vi "Teleop.vi"(10 "Match Info":T1={"Autonomous Elapsed Seconds"=0.0, "TeleOp Elapsed Seconds"=0.0, "Disabled Elapsed Seconds"=0.0, "Visited Autonomous"=FALSE, "Visited TeleOp"=FALSE, "Visited Disabled"=FALSE, "Autonomous Settings"={"Autonomous Style"=enum."Independent", "VI Refnum"=refnum}}, 11 "Call Context":T2) -> ()   [LabVIEW 2011]
doc: "This VI is called for each TeleOp packet received from the DS where the robot is not disabled. It is often used to read from the joysticks and update I/O or to update setpoints for timed control loops. It should complete and return within 20 milliseconds or it may miss DS packets."
uses:
  <vilib>/Rock Robotics/WPI/DriverStation/WPI_DriverStationDerivedRobotMode.ctl
  <vilib>/Rock Robotics/WPI/DriverStation/WPI_DriverStationMatch Info.ctl
  Robot Global Data.vi
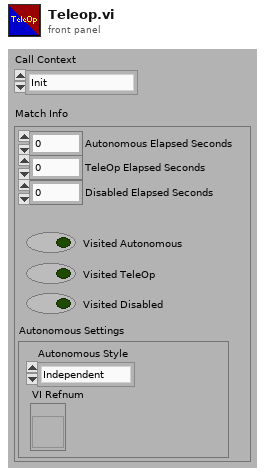
[diagram p1: front panel]
types:
  T1 = typedef "WPI_DriverStationMatch Info.ctl" = cluster{"Autonomous Elapsed Seconds":dbl, "TeleOp Elapsed Seconds":dbl, "Disabled Elapsed Seconds":dbl, "Visited Autonomous":bool, "Visited TeleOp":bool, "Visited Disabled":bool, "Autonomous Settings":cluster{"Autonomous Style":enum16{"Iterative", "Independent"}, "VI Refnum":refnum<vi>}}
  T2 = typedef "WPI_DriverStationDerivedRobotMode.ctl" = enum16{"Init", "Execute", "Stop"}
  T3 = typedef "WPI_RobotDriveDevRef.ctl" = cluster{"DevStatus":errorcluster, "Motors[]":T4[], "Square Inputs":bool, "Max Output":dbl, "Isochronous":bool}
  T4 = typedef "WPI_MotorControlDeviceRef.ctl" = cluster{"DeviceStatus":errorcluster, "Type":enum16{"PWM", "CAN"}, "PWM":cluster{"Digital Module":T5, "PWM Channel":T6, "DeadBand":T7}, "CAN":cluster{"Device Number":u8, "Control Mode":T8, "Semaphore":T9, "Max Vout":dbl}, "Invert":bool, "TransformRef":T10, "InvTransformRef":T10}
  T5 = typedef "FPGA_TypedefDigitalModule.ctl" = enum16{"Digital Module 1", "Digital Module 2"}
  T6 = typedef "FPGA_DIOPWMChannel.ctl" = enum8{"PWM 1", "PWM 2", "PWM 3", "PWM 4", "PWM 5", "PWM 6", "PWM 7", "PWM 8", "PWM 9", "PWM 10", "Invalid"}
  T7 = typedef "WPI_PWMDeadband.ctl" = cluster{"Name":string, "maxPositivePwm":i32, "minPositivePwm":i32, "centerPwm":i32, "maxNegativePwm":i32, "minNegativePwm":i32, "angularRange":u16}
  T8 = typedef "WPI_CANJaguar_ControlMode.ctl" = enum8{"Percent VBus", "Current", "Speed", "Position", "Voltage"}
  T9 = typedef "Semaphore RefNum" = refnum<k1>
  T10 = typedef "WPI_PWMTransform_ConPane.ctl" = refnum<vi>
  T11 = typedef "WPI_JoystickDevRef.ctl" = cluster{"Device":T12}
  T12 = typedef "WPI_JoystickDeviceEnum.ctl" = enum16{"USB 1", "USB 2", "USB 3", "USB 4", "Kinect 1", "Kinect 2"}
  T13 = typedef "WPI_JoystickButtonState.ctl" = cluster{"Button 1":bool, "Button 2":bool, "Button 3":bool, "Button 4":bool, "Button 5":bool, "Button 6":bool, "Button 7":bool, "Button 8":bool, "Button 9":bool, "Button 10":bool, "Button 11":bool, "Button 12":bool}
  T14 = cluster{"axis 1 (x)":dbl, "axis 2 (y)":dbl, "axis 3 (throttle)":dbl, "axis 4":dbl, "axis 5":dbl, "axis 6":dbl}
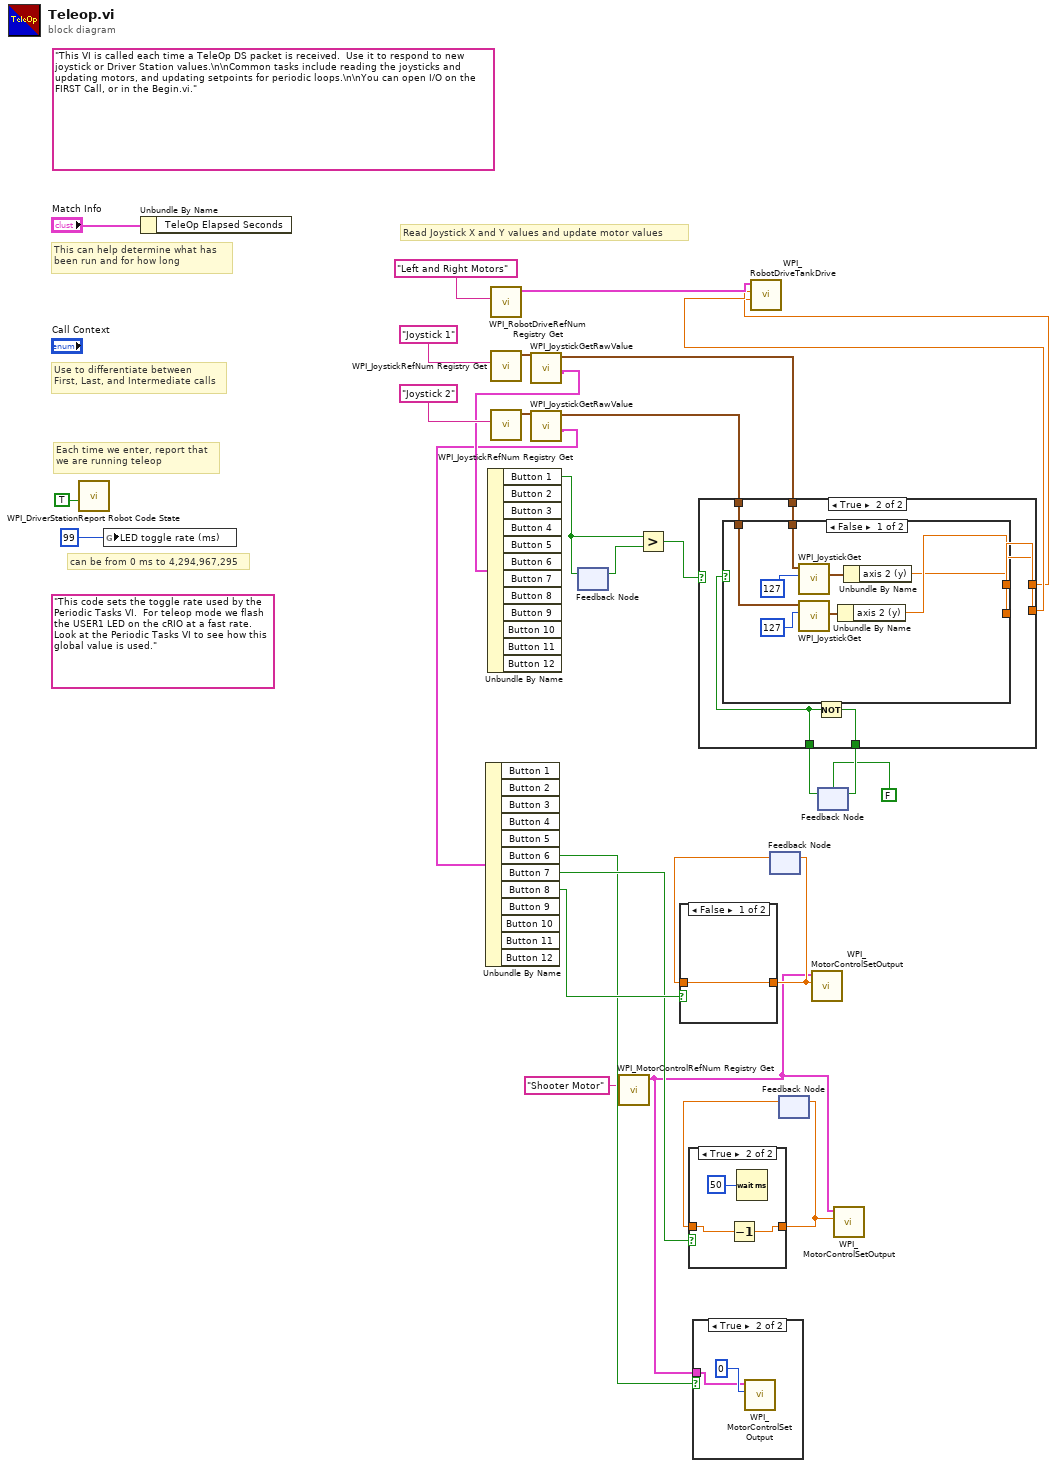
[diagram p0: block diagram]
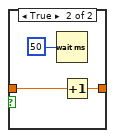
[diagram p4: hidden frame]
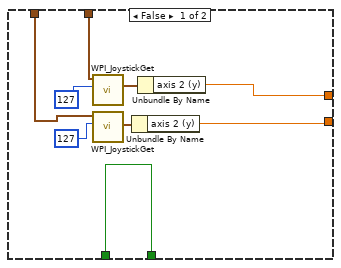
[diagram p5: hidden frame]
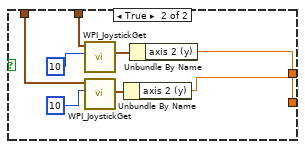
[diagram p6: hidden frame]
diagram:
  (unwired) "This code sets the toggle rate used by the Periodic Tasks VI.  For teleop mode we flash the USER1 LED on the cRIO at a fast rate.  Look at the Periodic Tasks VI to see how this global value is used."
  (unwired) "This VI is called each time a TeleOp DS packet is received.  Use it to respond to new joystick or Driver Station values.\n\nCommon tasks include reading the joysticks and updating motors, and updating setpoints for periodic loops.\n\nYou can open I/O on the FIRST Call, or in the Begin.vi."
  # "can be from 0 ms to 4,294,967,295"
  # "Each time we enter, report that\nwe are running teleop"
  # "Use to differentiate between\nFirst, Last, and Intermediate calls"
  # "This can help determine what has\nbeen run and for how long"
  # "Read Joystick X and Y values and update motor values"
  n1 = call <vilib>:"WPI_DriverStationReport Robot Code State.vi"("TeleOp"=TRUE ("Autonomous")) -> ()  [unwired: 10 in, 1 out]
  n2 = global write "Robot Global Data.vi" "LED toggle rate (ms)"(u32 99 ("LED ms toggle rate")) -> ()
  n3 = Unbundle By Name("Match Info") -> ()  [unwired: 1 out]
  n4 = call <vilib>:"WPI_RobotDriveRefNum Registry Get.vi"("refnum name"="Left and Right Motors") -> ("RobotDriveDevRef"=w25:T3)  [unwired: 1 in, 9 out]
  n5 = call <vilib>:"WPI_JoystickRefNum Registry Get.vi"("refnum name"="Joystick 1") -> ("JoystickDevRef"=w17:T11)  [unwired: 1 in, 9 out]
  n6 = call <vilib>:"WPI_JoystickRefNum Registry Get.vi"("refnum name"="Joystick 2") -> ("JoystickDevRef"=w15:T11)  [unwired: 1 in, 9 out]
  n7 = call <vilib>:"WPI_JoystickGetRawValue.vi"("JoystickDevRef"=w17) -> ("Buttons"=w16:T13, "JoystickDevRef"=w11:T11)  [unwired: 8 in, 1 out]
  n8 = Unbundle By Name(w16) -> ("Button 1"=w18:bool)  [unwired: 11 out]
  n9 = call <vilib>:"WPI_JoystickGetRawValue.vi"("JoystickDevRef"=w15) -> ("Buttons"=w14:T13, "JoystickDevRef"=w10:T11)  [unwired: 8 in, 1 out]
  n10 = Unbundle By Name(w14) -> ("Button 6"=w4:bool, "Button 7"=w5:bool, "Button 8"=w9:bool)  [unwired: 9 out]
  n11 = feedback #1() -> (w19:bool)  [unwired: 1 in]
  n12 = feedback-in #1(w18) -> ()
  n13 = call <vilib>:"WPI_MotorControlRefNum Registry Get.vi"("refnum name"="Shooter Motor") -> ("MotorControlDevRef"=w1:T4)  [unwired: 9 in, 1 out]
  n14 = Greater?(x=w18, y=w19) -> (0:w23:bool)
  n15 = case shown="True" w4 {
    tunnel: w1 -> [_ w31]
    frame False {
    }
    frame True {
      n16 = call <vilib>:"WPI_MotorControlSetOutput.vi"("Output"=0, "MotorControlDevRef"=w31) -> ()  [unwired: 8 in, 2 out]
    }
  }
  n17 = feedback #2() -> (w7:dbl)  [unwired: 1 in]
  n18 = case shown="False" w9 {
    tunnel: [w33 w36] -> w8
    tunnel: w7 -> [w33 w35]
    frame False {
    }
    frame True {
      n19 = Wait (ms)(milliseconds to wait=50) -> ()  [unwired: 1 out]
      n20 = Increment(x=w35) -> (x+1=w36:dbl)
    }
  }
  n21 = feedback-in #2(w8) -> ()
  n22 = feedback #3() -> (w6:dbl)  [unwired: 1 in]
  n23 = case shown="True" w5 {
    tunnel: [w37 w39] -> w2
    tunnel: w6 -> [w37 w38]
    frame False {
    }
    frame True {
      n24 = Decrement(x=w38) -> (x-1=w39:dbl)
      n25 = Wait (ms)(milliseconds to wait=50) -> ()  [unwired: 1 out]
    }
  }
  n26 = feedback-in #3(w2) -> ()
  n27 = call <vilib>:"WPI_MotorControlSetOutput.vi"("Output"=w8, "MotorControlDevRef"=w1) -> ()  [unwired: 8 in, 2 out]
  n28 = feedback #4(FALSE) -> (w22:bool)
  n29 = case shown="True" w23 {
    tunnel: w22 -> [w49 w54]
    tunnel: [w49 w55] -> w21
    tunnel: [w43 w53] -> w12
    tunnel: [w44 w52] -> w13
    tunnel: w11 -> [w42 w51]
    tunnel: w10 -> [w41 w50]
    frame False {
      n30 = call <vilib>:"WPI_JoystickGet.vi"("Scaler"=127, "JoystickDevRef"=w42) -> ("Axes"=w48:T14)  [unwired: 5 out]
      n31 = call <vilib>:"WPI_JoystickGet.vi"("Scaler"=127, "JoystickDevRef"=w41) -> ("Axes"=w47:T14)  [unwired: 5 out]
      n32 = Unbundle By Name(w47) -> ("axis 2 (y)"=w44:dbl)
      n33 = Unbundle By Name(w48) -> ("axis 2 (y)"=w43:dbl)
    }
    frame True {
      n34 = case shown="False" w54 {
        tunnel: [w58 w69] -> w53
        tunnel: [w59 w68] -> w52
        tunnel: w51 -> [w57 w65]
        tunnel: w50 -> [w56 w64]
        frame False {
          n35 = call <vilib>:"WPI_JoystickGet.vi"("Scaler"=127, "JoystickDevRef"=w57) -> ("Axes"=w60:T14)  [unwired: 5 out]
          n36 = call <vilib>:"WPI_JoystickGet.vi"("Scaler"=127, "JoystickDevRef"=w56) -> ("Axes"=w61:T14)  [unwired: 5 out]
          n37 = Unbundle By Name(w61) -> ("axis 2 (y)"=w59:dbl)
          n38 = Unbundle By Name(w60) -> ("axis 2 (y)"=w58:dbl)
        }
        frame True {
          n39 = call <vilib>:"WPI_JoystickGet.vi"("Scaler"=10, "JoystickDevRef"=w65) -> ("Axes"=w71:T14)  [unwired: 5 out]
          n40 = call <vilib>:"WPI_JoystickGet.vi"("Scaler"=10, "JoystickDevRef"=w64) -> ("Axes"=w70:T14)  [unwired: 5 out]
          n41 = Unbundle By Name(w70) -> ("axis 2 (y)"=w68:dbl)
          n42 = Unbundle By Name(w71) -> ("axis 2 (y)"=w69:dbl)
        }
      }
      n43 = Not(x=w54) -> (.not. x?=w55:bool)
    }
  }
  n44 = call <vilib>:"WPI_RobotDriveTankDrive.vi"("Right axis value"=w12, "Left axis value"=w13, "RobotDriveDevRef"=w25) -> ()  [unwired: 7 in, 2 out]
  n45 = feedback-in #4(w21) -> ()
  n46 = call <vilib>:"WPI_MotorControlSetOutput.vi"("Output"=w2, "MotorControlDevRef"=w1) -> ()  [unwired: 8 in, 2 out]
